vi "ARM MACROS.vi"(8 "error in (no error)":errorcluster, 10 "Array":T2(array[cluster]) {"RIGHT"."Angle"."speed" min=0.0 max=1.0 format="%_3g"; "RIGHT"."Angle"."ARM ANGLE (deg)" format="%.3g"; "RIGHT"."Climber"."CLIMBER STROKE (in)" format="%_5g"; "RIGHT"."Climber"."speed" min=0.0 max=1.0 format="%_3g"; "LEFT"."Angle"."speed" min=0.0 max=1.0 format="%_3g"; "LEFT"."Angle"."ARM ANGLE (deg)" format="%.3g"; "LEFT"."Climber"."CLIMBER STROKE (in)" format="%_5g"; "LEFT"."Climber"."speed" min=0.0 max=1.0 format="%_3g"}) -> (0 "error out":errorcluster)   [LabVIEW 2020]
uses:
  ctrl ARM MACRO ENTRY.ctl
  <vilib>/Rock Robotics/Network Tables/NT Write String.vi
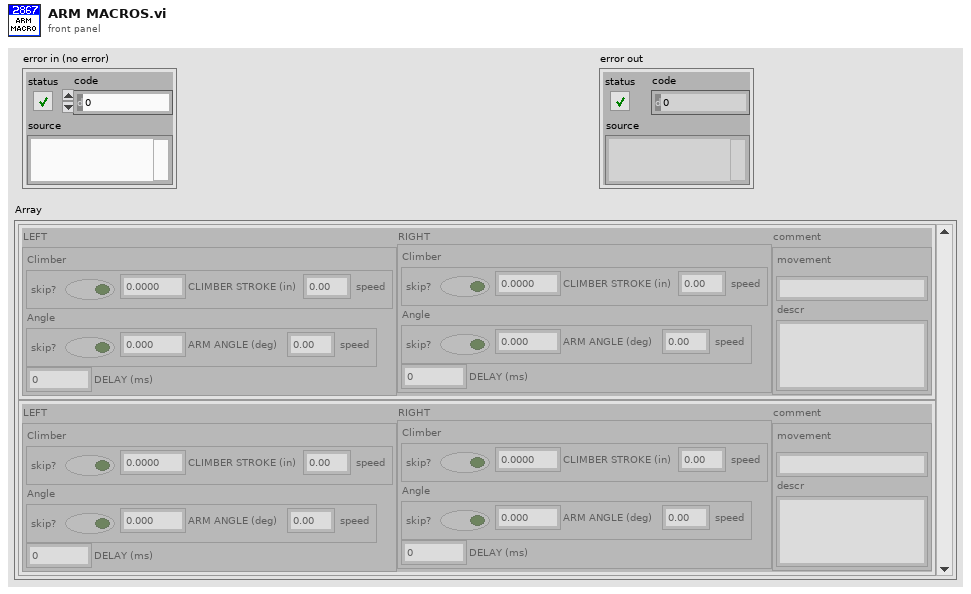
[diagram p1: front panel]
types:
  T1 = typedef "ctrl ARM MACRO ENTRY.ctl" = cluster{"Climber":cluster{"skip?":bool, "CLIMBER STROKE (in)":dbl, " speed":dbl}, "Angle":cluster{"skip?":bool, "ARM ANGLE (deg)":dbl, " speed":dbl}, "DELAY (ms)":u32}
  T2 = cluster{"LEFT":T1, "RIGHT":T1, "comment":cluster{"movement":string, "descr":string}}[]
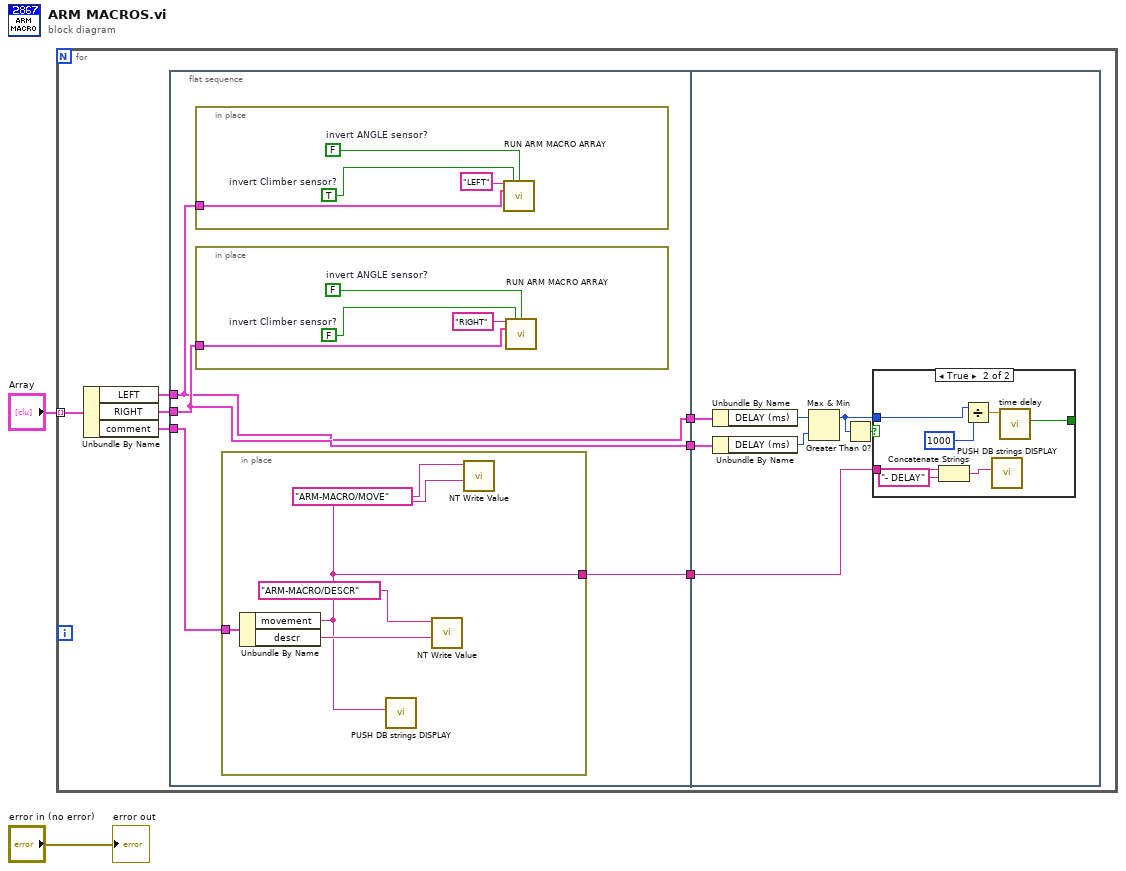
[diagram p0: block diagram]
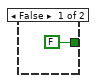
[diagram p2: hidden frame]
diagram:
  n1 = for {
    tunnel: "Array" -> [w9] mode=indexing
    n2 = Unbundle By Name(w9) -> ("LEFT"=w8:T1, "RIGHT"=w7:T1, "comment"=w4:cluster{"movement":string, "descr":string})
    n3 = flat-sequence {
      tunnel: w8 -> [w12]
      tunnel: w7 -> [w13]
      tunnel: [w13] -> w6
      tunnel: [w12] -> w5
      tunnel: w4 -> [w11]
      tunnel: [w10] -> w3
      tunnel: w6 -> [w32]
      tunnel: w5 -> [w28]
      tunnel: w3 -> [w27]
      frame #0 {
        n4 = in-place {
          in-place-border: w12 -> [w23]
          w26 = TRUE  # invert Climber sensor?
          w25 = FALSE  # invert ANGLE sensor?
          n5 = call "RUN ARM MACRO ARRAY.vi"("LEFT or RIGHT"="LEFT" ("String"), "invert Climber sensor?"=w26, "invert ANGLE sensor?"=w25, "element of ARRAY ROW"=w23) -> ()  [unwired: 12 in]
        }
        n6 = in-place {
          in-place-border: w13 -> [w19]
          w22 = FALSE  # invert Climber sensor?
          w21 = FALSE  # invert ANGLE sensor?
          n7 = call "RUN ARM MACRO ARRAY.vi"("LEFT or RIGHT"="RIGHT" ("String"), "invert Climber sensor?"=w22, "invert ANGLE sensor?"=w21, "element of ARRAY ROW"=w19) -> ()  [unwired: 12 in]
        }
        n8 = in-place {
          in-place-border: w11 -> [w17]
          in-place-border: [w14] -> w10
          n9 = Unbundle By Name(w17) -> ("movement"=w14:string, "descr"=w16:string)
          n10 = call "PUSH DB strings DISPLAY.vi"("NEW String"=w14) -> ()  [unwired: 10 in, 1 out]
          n11 = call-poly <vilib>:"NT Write Value.vi"("String"=w16, "Name"="ARM-MACRO/DESCR") -> ()  [unwired: 9 in, 1 out]
          n12 = call-poly <vilib>:"NT Write Value.vi"("String"=w14, "Name"="ARM-MACRO/MOVE") -> ()  [unwired: 9 in, 1 out]
        }
      }
      frame #1 {
        n13 = Unbundle By Name(w28) -> ("DELAY (ms)"=w29:u32)
        n14 = Unbundle By Name(w32) -> ("DELAY (ms)"=w30:u32)
        n15 = Max & Min(x=w29, y=w30) -> (max(x,y)=w31:u32)  [unwired: 1 out]
        n16 = Greater Than 0?(x=w31) -> (x > 0?=w33:bool)
        n17 = case shown="True" w33 {
          tunnel: w31 -> [_ w36]
          tunnel: [FALSE ("done?") w40] -> _
          tunnel: w27 -> [_ w39]
          frame False {
          }
          frame True {
            n18 = Concatenate Strings(w39, "- DELAY" ("string")) -> (w38:string)
            n19 = Divide(x=w36, y=u32 1000 ("x")) -> (x/y=w41:dbl)
            n20 = call "PUSH DB strings DISPLAY.vi"("NEW String"=w38) -> ()  [unwired: 10 in, 1 out]
            n21 = call "time delay.vi"("timer delay (s)"=w41) -> ("done?"=w40:bool)  [unwired: 9 in, 1 out]
          }
        }
      }
    }
  }
  "error out" <- "error in (no error)"
